vi "GatherChannelDataForGraph.vi"(8 "error in (no error)":errorcluster, 10 "Channel (-1 for all)":i64, 11 "OXY_SCPI Reseource In":refnum<visa-resource-name>) -> (0 "error out":errorcluster, 2 "Data":T1[](array[typedef]), 3 "OXY_SCPI Reseource Out":refnum<visa-resource-name>)   [LabVIEW 2018, in "OXYGEN.lvlib"]
uses:
  OXYGEN.lvlib
  TypeDefs/SingleDataElement.ctl
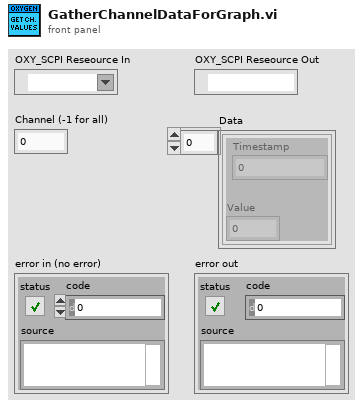
[diagram p1: front panel]
types:
  T1 = typedef "SingleDataElement.ctl" = cluster{"Timestamp":dbl, "Value":dbl}
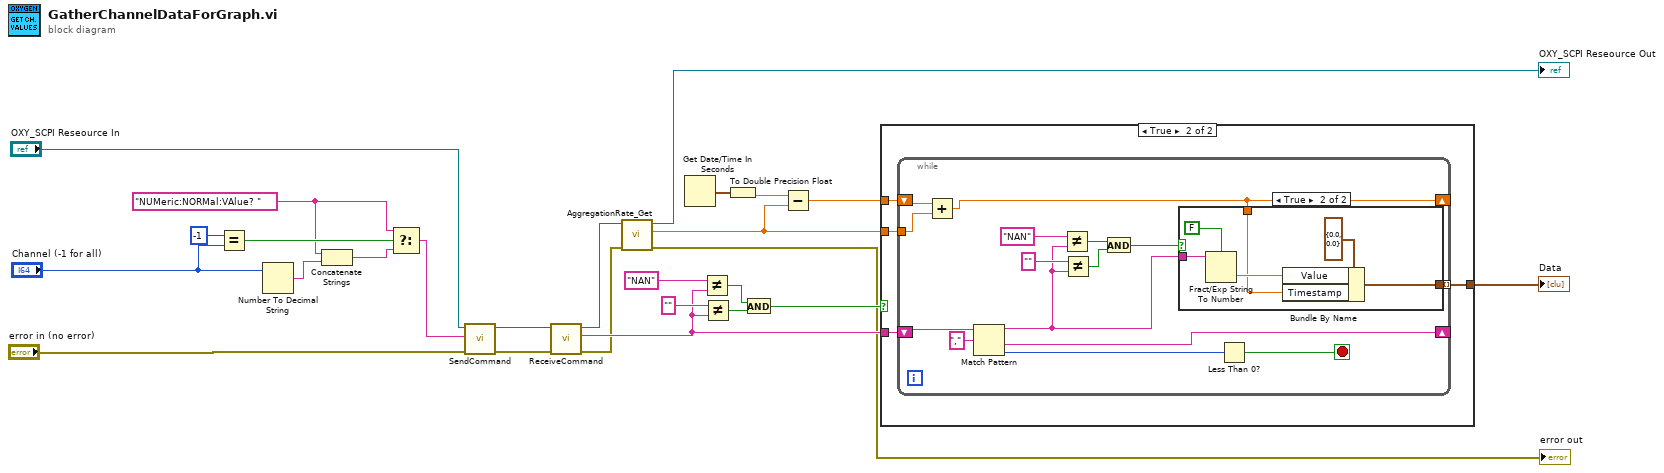
[diagram p0: block diagram]
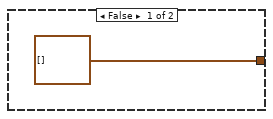
[diagram p2: hidden frame]
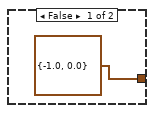
[diagram p3: hidden frame]
diagram:
  w2 = "NUMeric:NORMal:VAlue? " ("string")
  n1 = Equal?(x=i64 -1, y="Channel (-1 for all)") -> (x = y?=w4:bool)
  n2 = Number To Decimal String(number="Channel (-1 for all)") -> (decimal integer string=w12:string)  [unwired: 1 in]
  n3 = Concatenate Strings(w2, w12) -> (w3:string)
  n4 = Select(t=w2, s=w4, f=w3) -> (s? t:f=w1:string)
  n5 = call "SendCommand.vi"("error in (no error)"="error in (no error)", "String to Send"=w1, "OXY_SCPI Reseource In"="OXY_SCPI Reseource In") -> ("error out"=w8:errorcluster, "OXY_SCPI Reseource Out"=w11:refnum<visa-resource-name>)  [unwired: 7 in]
  n6 = call "ReceiveCommand.vi"("error in (no error)"=w8, "OXY_SCPI Reseource In"=w11) -> ("error out"=w9:errorcluster, "received Data"=w13:string, "OXY_SCPI Reseource Out"=w10:refnum<visa-resource-name>)  [unwired: 6 in, 1 out]
  n7 = call "AggregationRate_Get.vi"("error in (no error)"=w9, "OXY_SCPI Reseource In"=w10) -> ("error out"=→"error out":errorcluster, "Rate (s)"=w21:dbl, "OXY_SCPI Reseource Out"=→"OXY_SCPI Reseource Out":refnum<visa-resource-name>)  [unwired: 6 in, 1 out]
  n8 = Get Date/Time In Seconds() -> (seconds since 1Jan1904=w23:timestamp)
  n9 = Not Equal?(x="NAN", y=w13) -> (x != y?=w16:bool)
  n10 = Not Equal?(x="", y=w13) -> (x != y?=w17:bool)
  n11 = To Double Precision Float(number=w23) -> (double precision float=w22:dbl)
  n12 = And(x=w16, y=w17) -> (x .and. y?=w15:bool)
  n13 = Subtract(x=w22, y=w21) -> (x-y=w20:dbl)
  n14 = case shown="True" w15 {
    tunnel: w13 -> [_ w31]
    tunnel: [T1[] [] w30] -> w25
    tunnel: w21 -> [_ w29]
    tunnel: w20 -> [_ w28]
    frame False {
    }
    frame True {
      n15 = while {
        shift-right: [w44] -> _
        shift-left: w31 -> [w46]
        tunnel: [w41] -> w30 mode=indexing
        shift-right: [w38] -> _
        shift-left: w28 -> [w40]
        tunnel: w29 -> [w39]
        stop <- w42 stop-if-true
        n16 = Add(x=w40, y=w39) -> (x+y=w38:dbl)
        n17 = Match Pattern(string=w46, regular expression=",") -> (before substring=w33:string, after substring=w44:string, offset past match=w43:i32)  [unwired: 1 in, 1 out]
        n18 = Not Equal?(x="NAN", y=w33) -> (x != y?=w34:bool)
        n19 = Not Equal?(x="", y=w33) -> (x != y?=w35:bool)
        n20 = And(x=w34, y=w35) -> (x .and. y?=w32:bool)
        n21 = case shown="True" w32 {
          tunnel: [T1 {"Timestamp"=-1.0, "Value"=0.0} w51] -> w41
          tunnel: w38 -> [_ w50]
          tunnel: w33 -> [_ w49]
          frame False {
          }
          frame True {
            n22 = Fract/Exp String To Number(use system decimal point (T)=FALSE, string=w49) -> (number=w53:dbl)  [unwired: 2 in, 1 out]
            n23 = Bundle By Name(cluster=T1 {"Timestamp"=0.0, "Value"=0.0}, "Value"=w53, "Timestamp"=w50) -> (w51:T1)
          }
        }
        n24 = Less Than 0?(x=w43) -> (x < 0?=w42:bool)
      }
    }
  }
  "Data" <- w25
